vi "SQL Results to Trace.vi"(8 "error in (no error)":errorcluster, 9 "Result":string[][](array[string]), 10 "PG Path":string, 11 "Database Viewer":refnum<class "Database Viewer.lvclass">) -> (0 "error out":errorcluster, 1 "Latest Value":string, 2 "Trace":cluster{timestamp[], dbl[]}, 3 "Database Viewer out":refnum<class "Database Viewer.lvclass">)   [LabVIEW 2019, in "Database Viewer.lvclass"]
uses:
  Database Viewer.lvclass
  <userlib>/LevyLab/LV-Data/LV-Data.PG/LV-Data.PGSQL.lvclass
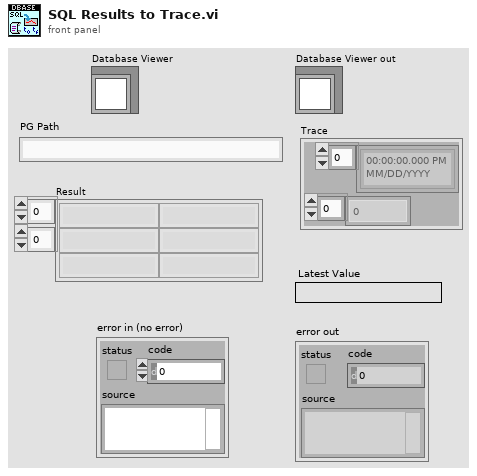
[diagram p1: front panel]
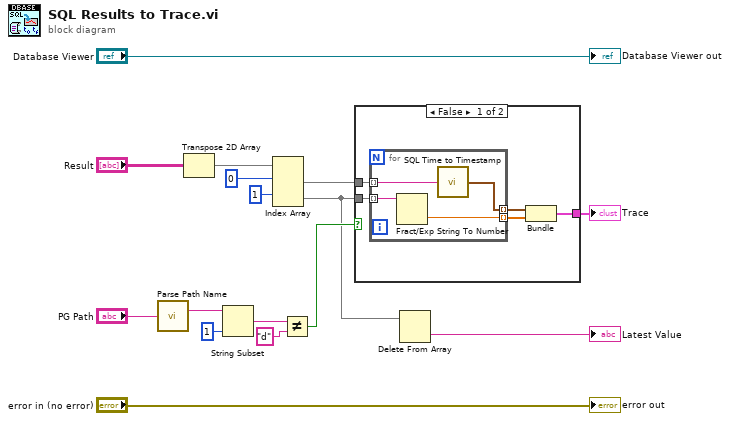
[diagram p0: block diagram]
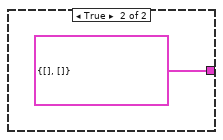
[diagram p2: hidden frame]
diagram:
  n1 = call <userlib>:"Parse Path Name.vi"("PG Path"="PG Path") -> ("Column path"=w6:string)  [unwired: 10 in, 4 out]
  n2 = Transpose 2D Array(2D array="Result") -> (transposed array=w13:string[][])
  n3 = String Subset(string=w6, length (rest)=1 ("length (rest)")) -> (substring=w8:string)  [unwired: 1 in]
  n4 = Index Array(array=w13, index (row) #1=0 ("index (row)"), index (row) #2=1 ("index (row)")) -> (element #1=w16:string[], element #2=w3:string[])  [unwired: 2 in]
  n5 = Not Equal?(x=w8, y="d") -> (x != y?=w4:bool)
  n6 = case shown="False" w4 {
    tunnel: w3 -> [w19 _]
    tunnel: w16 -> [w18 _]
    tunnel: [w17 cluster{timestamp[], dbl[]} {[], []}] -> w11
    frame False {
      n7 = for {
        tunnel: w18 -> [w23] mode=indexing
        tunnel: w19 -> [w25] mode=indexing
        tunnel: [w24] -> w21 mode=indexing
        tunnel: [w22] -> w20 mode=indexing
        n8 = Fract/Exp String To Number(string=w25) -> (number=w24:dbl)  [unwired: 3 in, 1 out]
        n9 = call "SQL Time to Timestamp.vi"("Get:Get String"=w23) -> ("Time Stamp"=w22:timestamp)
      }
      n10 = Bundle(w20, w21) -> (w17:cluster{timestamp[], dbl[]})  [unwired: 1 in]
    }
    frame True {
    }
  }
  "Trace" <- w11
  n11 = Delete From Array(array=w3) -> (deleted portion=→"Latest Value":string)  [unwired: 2 in, 1 out]
  "error out" <- "error in (no error)"
  "Database Viewer out" <- "Database Viewer"
